vi "DriveSetFeet.vi"(2 "Feet":dbl=10.0 format="%#_13g", 3 "Direction":T1(ring)) -> (0 "Rate (Rev/Sec)":dbl(knob) scale=0.0..100.0, 1 "Distance Travelled (Feet)":dbl(knob) scale=0.0..10.0)   [LabVIEW 2014]
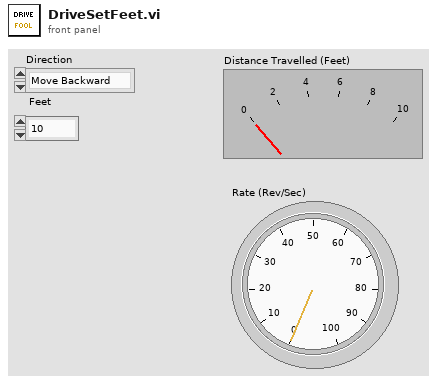
[diagram p1: front panel]
types:
  T1 = enum16{"Move Backward", "Move Forward", "Strafe Right", "Strafe Left"}
  T2 = cluster{"Distance":dbl, "Rate":dbl, "Direction":bool, "Stopped":bool}[]
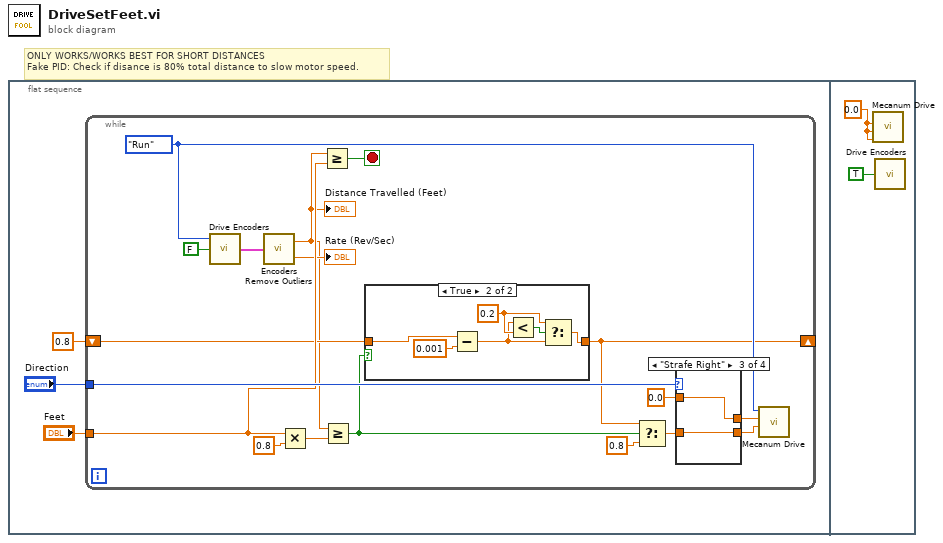
[diagram p0: block diagram]
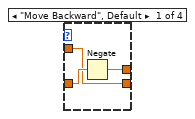
[diagram p3: hidden frame]
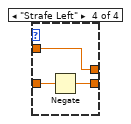
[diagram p5: hidden frame]
diagram:
  # "ONLY WORKS/WORKS BEST FOR SHORT DISTANCES\nFake PID: Check if disance is 80% total distance to slow motor speed."
  n1 = flat-sequence {
    frame #0 {
      n2 = while {
        tunnel: "Direction" -> [w19]
        tunnel: "Feet" -> [w14]
        shift-right: [w9] -> _
        shift-left: 0.8 -> [w10]
        stop <- w20 stop-if-true
        w17 = enum8{"Start", "Run", "Finish"}."Run" ("Mode")
        n3 = call "Drive Encoders.vi"("Reset"=FALSE, "Mode"=w17) -> ("Encoder"=w6:T2)  [unwired: 1 in]
        n4 = call "Encoders Remove Outliers.vi"("array"=w6) -> ("Mean Distance"=w4:dbl, "Mean Rate"=→"Rate (Rev/Sec)":dbl)
        "Distance Travelled (Feet)" <- w4
        n5 = Multiply(x=w14, y=0.8) -> (x*y=w12:dbl)
        n6 = Greater Or Equal?(x=w4, y=w14) -> (x >= y?=w20:bool)
        n7 = Greater Or Equal?(x=w4, y=w12) -> (x >= y?=w8:bool)
        n8 = case shown="True" w8 {
          tunnel: w10 -> [w22 w27]
          tunnel: [w22 w23] -> w9
          frame False {
          }
          frame True {
            w25 = 0.2 ("y")
            n9 = Subtract(x=w27, y=0.001) -> (x-y=w24:dbl)
            n10 = Less?(x=w24, y=w25) -> (x < y?=w26:bool)
            n11 = Select(t=w25, s=w26, f=w24) -> (s? t:f=w23:dbl)
          }
        }
        n12 = Select(t=w9, s=w8, f=0.8) -> (s? t:f=w7:dbl)
        n13 = case shown="\"Strafe Right\"" w19 {
          tunnel: w7 -> [w31 w33 w35 w38]
          tunnel: [w30 w33 w34 w36] -> w18
          tunnel: [w29 w32 w35 w37] -> w16
          tunnel: 0.0 ("Turn") -> [w29 w32 w34 w36]
          frame "Move Backward", Default {
            n14 = Negate(x=w31) -> (-x=w30:dbl)
          }
          frame "Move Forward" {
          }
          frame "Strafe Right" {
          }
          frame "Strafe Left" {
            n15 = Negate(x=w38) -> (-x=w37:dbl)
          }
        }
        n16 = call "Mecanum Drive.vi"("Strafe"=w16, "Forward/Backward"=w18, "Mode"=w17) -> ()  [unwired: 9 in]
      }
    }
    frame #1 {
      w40 = 0.0 ("Forward/Backward")
      n17 = call "Mecanum Drive.vi"("Turn"=w40, "Strafe"=w40, "Forward/Backward"=w40) -> ()  [unwired: 9 in]
      n18 = call "Drive Encoders.vi"("Reset"=TRUE) -> ()  [unwired: 2 in, 1 out]
    }
  }
